vi "OE2052_USB_Query Data.vi"(0 "VISA resource name":refnum<visa-resource-name>, 11 "Error in (no error)":errorcluster caption="error out（no error）") -> (3 "Buffer Count":u8, 4 "VISA resource  out":refnum<visa-resource-name>, 6 "Parameter Values":T2, 8 "Total Data Array":dbl[][](array[numeric]), 10 "Output String":string, 14 "A&B_PLL&Overload":T1, 15 "Error out":errorcluster caption="error out")   [LabVIEW 2011]
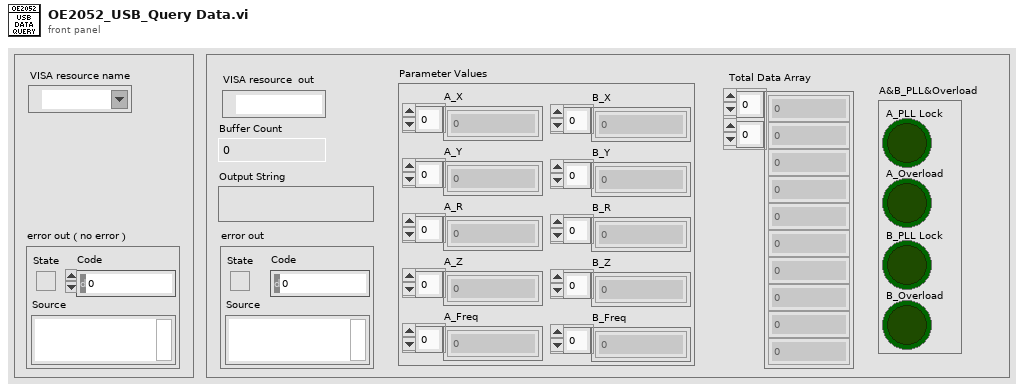
[diagram p1: front panel]
types:
  T1 = cluster{"A_PLL Lock":bool, "A_Overload":bool, "B_PLL Lock":bool, "B_Overload":bool}
  T2 = cluster{"A_X":dbl[], "A_Y":dbl[], "A_R":dbl[], "A_Z":dbl[], "A_Freq":dbl[], "B_X":dbl[], "B_Y":dbl[], "B_R":dbl[], "B_Z":dbl[], "B_Freq":dbl[]}
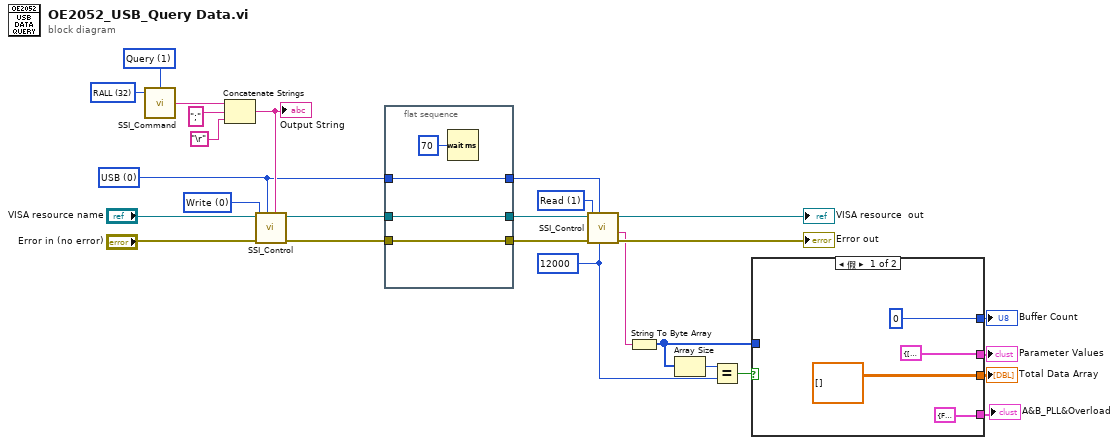
[diagram p0: block diagram]
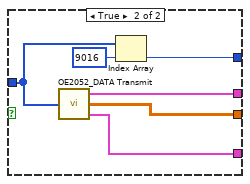
[diagram p2: hidden frame]
diagram:
  w2 = u16 0 items=["USB"=0, "RS232"=1, "Ethernet"=3] ("Remote Mode")
  w14 = u32 12000 ("Number of bytes")
  w17 = u16 1 items=["Write", "Read"] ("Control")
  w19 = u16 0 items=["Write", "Read"] ("Control")
  w24 = u16 32 items=["ISRC", "IGND", "ICPL", "ILIN", "PHAS", "FMOD", "RSLP", "FREQ", "SWPT", "SLLM", "SULM", "SSLL", "SSLG", "STLM", "SWRM", "IRNG", "SENS", "RMOD", "OFLT", "OFSL", "SYNC", "DMOD", "HARM", "DARB", "SWVT", "SLVL", "SVLL", "SVUL", "SVSL", "SVSG", "SVTM", "SVRM", "RALL", "SNAP", "OUTP", "OAUX", "COUT", "CAUX", "COFP", "CEXP", "FPOP", "OEXP", "*IDN", "*RST", "OVLD", "INOV", "GNOV", "*PLL", "SSET", "RSET", "AGAN", "APHS", "ARSV", "ASCL", "EQCD", "EQCS", "SPED", "SRAT", "SLEN", "SSLE", "STRG", "SPRM", "STRD", "PAUS", "RSET", "SPTS", "TRCA", "TEMP", "RSTU", "INHZ", "DEQU", "SADD", "ARNG", "CSPE", "ISRCD", "IGNDD", "ICPLD", "ILIND", "PHASD", "FMODD", "RSLPD", "FREQD", "SWPTD", "SLLMD", "SULMD", "SSLLD", "SSLGD", "STLMD", "SWRMD", "SENSD", "RMODD", "OFLTD", "OFSLD", "SYNCD", "HARMD", "EQCDD", "EQCSD", "SNAPD", "OUTPD", "SWVTD", "SLVLD", "SVLLD", "SVULD", "SVSLD", "SVSGD", "SVTMD", "SVRMD", "SVDCD", "ARSVD", "AGAND", "APHSD", "ASCLD", "FPOPD", "CAUXD", "OEXPD", "SPEDD", "SRATD", "SLEND", "SSLED", "STRGD", "SPRMD", "STRDD", "PAUSD", "RESTD", "SPTSD", "TRCAD", "*IDND", "*RSTD", "INOVD", "GNOVD", "*PLLD", "SSETD", "RSETD", "RALLD"] ("Command Type")
  w22 = u16 1 items=["Set", "Query"] ("Opera")
  n1 = call "SSI_Command.vi"("Opera"=w22, "Command Type"=w24) -> ("Output string"=w25:string)  [unwired: 2 in]
  n2 = Concatenate Strings(w25, ";" ("字符串"), "\r") -> (w27:string)
  "Output String" <- w27
  n3 = call "SSI_Control.vi"("Write Buffer"=w27, "Remote Mode"=w2, "Error in (no error)"="Error in (no error)", "Control"=w19, "VISA resource name"="VISA resource name") -> ("Error out"=w7:errorcluster, "VISA resource  out"=w8:refnum<visa-resource-name>)  [unwired: 3 in, 2 out]
  n4 = flat-sequence {
    tunnel: [w30] -> w9
    tunnel: w2 -> [w30]
    tunnel: [w29] -> w5
    tunnel: w8 -> [w29]
    tunnel: [w28] -> w6
    tunnel: w7 -> [w28]
    frame #0 {
      n5 = Wait (ms)(milliseconds to wait=u32 70 ("等待时间（毫秒）")) -> ()  [unwired: 1 out]
    }
  }
  n6 = call "SSI_Control.vi"("Number of bytes"=w14, "Remote Mode"=w9, "Error in (no error)"=w6, "Control"=w17, "VISA resource name"=w5) -> ("Error out"=→"Error out":errorcluster, "Read Buffer"=w15:string, "VISA resource  out"=→"VISA resource  out":refnum<visa-resource-name>)  [unwired: 3 in, 1 out]
  n7 = String To Byte Array(string=w15) -> (unsigned byte array=w10:u8[])
  n8 = Array Size(array=w10) -> (size(s)=w11:i32)
  n9 = Equal?(x=w11, y=w14) -> (x = y?=w12:bool)
  n10 = case shown="假" w12 {
    tunnel: [u8 0 w40] -> w13
    tunnel: w10 -> [_ w39]
    tunnel: [dbl[][] [] ("Total Data Array") w38] -> w4
    tunnel: [T2 {"A_X"=[], "A_Y"=[], "A_R"=[], "A_Z"=[], "A_Freq"=[], "B_X"=[], "B_Y"=[], "B_R"=[], "B_Z"=[], "B_Freq"=[]} ("Parameter Values") w37] -> w3
    tunnel: [T1 {"A_PLL Lock"=FALSE, "A_Overload"=FALSE, "B_PLL Lock"=FALSE, "B_Overload"=FALSE} ("A&B_PLL&Overload") w36] -> w1
    frame False {
    }
    frame True {
      n11 = call "OE2052_DATA Transmit.vi"("Input Data"=w39) -> ("Parameter Values"=w37:T2, "Total Data Array"=w38:dbl[][], "A&B_PLL&Overload"=w36:T1)
      n12 = Index Array(array=w39, index=9016 ("索引")) -> (element=w40:u8)
    }
  }
  "Buffer Count" <- w13
  "Parameter Values" <- w3
  "Total Data Array" <- w4
  "A&B_PLL&Overload" <- w1
